vi "Do That Thang Core.vi"(7 "Test Executive Ref out":refnum<data-value>, 8 "error in (no error)":errorcluster, 9 "Attributes Ref":refnum<data-value>, 11 "Device End Finder in":refnum<class "Device End Finder.lvclass">) -> (0 "error out":errorcluster)   [LabVIEW 2019, in "Nested Conditional in While Loop Example.lvlib" / "Device End Finder.lvclass"]
uses:
  <vilib>/gpm_packages/@cs/test-executive/Source/Sandbox/Nested Conditional in While Loop Example/Device End Finder/Device End Finder.lvclass
  <vilib>/gpm_packages/@cs/test-executive/Source/Test Executive/ITestExecutive/ITest Executive.lvclass
  <vilib>/gpm_packages/@cs/lookup-table/Source/LookupTable/LookupTable.lvclass
  <vilib>/gpm_packages/@cs/lookup-table/Source/LookupTable/LookupTable.lvclass/LookupTable.ctl
  f8aa2406-8f08-4b04-9a73-b68e01d5b8b9.vi
  629aea9d-b4c5-4a92-9ac2-79e49a526552.vi
  <vilib>/gpm_packages/@cs/lookup-table/Source/LookupTable/Read Table Reference.vi
  f8aa2406-8f08-4b04-9a73-b68e01d5b8b9.vi/4a39f1d6-fc73-43f9-b7a6-188aebfa0a55.vi
  <vilib>/Utility/error.llb/Error Cluster From Error Code.vi
  <vilib>/gpm_packages/@cs/test-executive/Source/Test Executive/TestExecutive Ref/TestExecutive Ref.lvclass
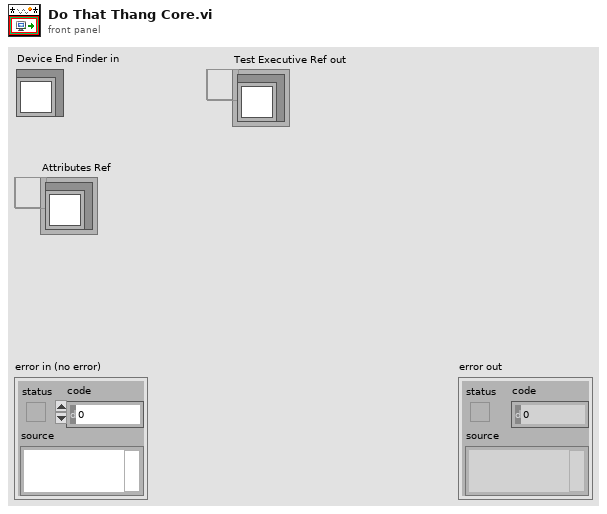
[diagram p1: front panel]
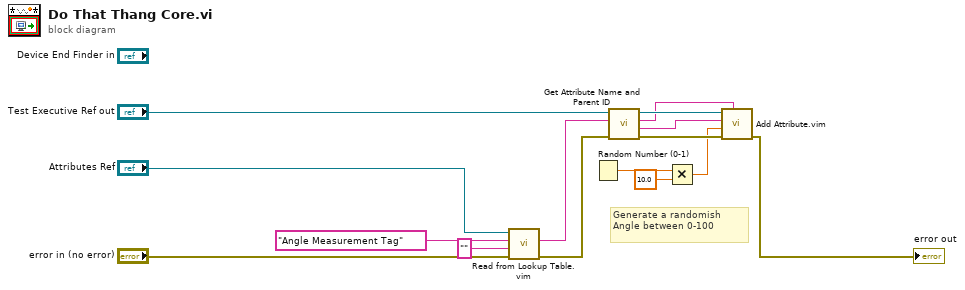
[diagram p0: block diagram]
diagram:
  # "Generate a randomish \nAngle between 0-100"
  n1 = call "Read from Lookup Table.vim"("error in (no error)"="error in (no error)", "Type"="", "Item Name"="Angle Measurement Tag", "LookupTable Reference"="Attributes Ref") -> ("error out"=w9:errorcluster, "Value"=w10:string)  [unwired: 4 in, 2 out]
  n2 = Random Number (0-1)() -> (number: 0 to 1=w4:dbl)
  n3 = call <vilib>:"Get Attribute Name and Parent ID.vi"("error in (no error)"=w9, "Tag"=w10, "Test Executive Ref"="Test Executive Ref out") -> ("error out"=w7:errorcluster, "Attribute Name"=w6:string, "Parent ID"=w5:string, "Test Executive Ref out"=w8:refnum<data-value>)  [unwired: 5 in]
  n4 = Multiply(x=w4, y=10.0) -> (x*y=w2:dbl)
  n5 = call "Add Attribute.vim"("ID"=w5, "error in (no error)"=w7, "Attribute"=w2, "Attribute Name"=w6, "Test Executive Ref"=w8) -> ("error out"=→"error out":errorcluster)  [unwired: 3 in, 3 out]
